vi "Un-Subscribe.vi"() -> ()   [LabVIEW 2013, in "FRCts20_SNS.lvlib"]
uses:
  FRCts20_SNS.lvlib
  Perforce/penguin_1666/mblack_PerforceWin/lvdotcom/source/aws-toolkit/r1/trunk/SNS/VI Source/AWS SNS Class/AWS_SNS.lvclass
  <vilib>/National Instruments/LabVIEW Interface for Amazon S3/Typedefs/AMZ_S3_AWS Credentials.ctl
  <vilib>/National Instruments/LabVIEW Interface for Amazon S3/LV Interface for Amazon S3.lvlib
  Perforce/penguin_1666/mblack_PerforceWin/lvdotcom/source/aws-toolkit/r1/trunk/SNS/VI Source/Public Typedefs/AWS_SNS Subcribe Parameters.ctl
  Perforce/penguin_1666/mblack_PerforceWin/lvdotcom/source/aws-toolkit/r1/trunk/SNS/VI Source/AWS_SNS.lvlib
  Perforce/penguin_1666/mblack_PerforceWin/lvdotcom/source/aws-toolkit/r1/trunk/SNS/VI Source/Public Typedefs/AWS_SNS Subscription.ctl
  Perforce/penguin_1666/mblack_PerforceWin/lvdotcom/source/aws-toolkit/r1/trunk/SNS/VI Source/Response Typedefs/ListSubscriptionsByTopicResult.ctl
panel:
  out "ListSubscriptions Result":T1
  in  "Event Name":string
  in  "Cell#":string
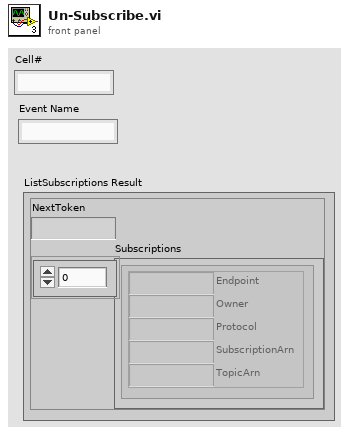
[diagram p1: front panel]
types:
  T1 = typedef "AWS_SNS.lvlib/ListSubscriptionsByTopicResult.ctl" = cluster{"NextToken":string, "Subscriptions":T2[]}
  T2 = typedef "AWS_SNS.lvlib/AWS_SNS Subscription.ctl" = cluster{"Endpoint":string, "Owner":string, "Protocol":string, "SubscriptionArn":string, "TopicArn":string}
  T3 = typedef "AWS_SNS.lvlib/AWS_SNS Subcribe Parameters.ctl" = cluster{"Endpoint":string, "Protocol":string, "TopicArn":string}
  T4 = typedef "LV Interface for Amazon S3.lvlib/AMZ_S3_AWS Credentials.ctl" = cluster{"Access Key":string, "Secret Key":string}
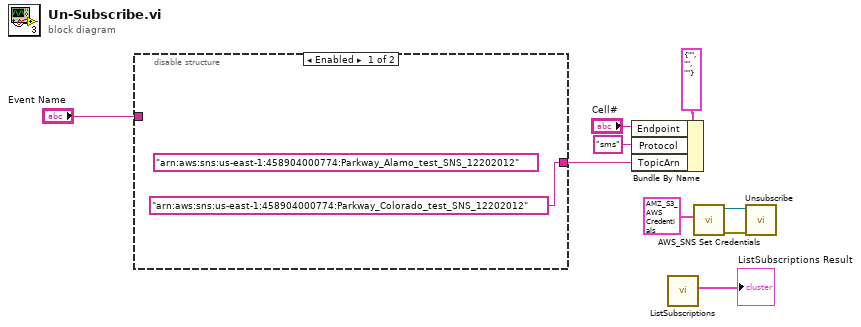
[diagram p0: block diagram]
diagram:
  n1 = disable-structure shown="Enabled" {
    disable-tunnel: ["arn:aws:sns:us-east-1:458904000774:Parkway_Colorado_test_SNS_12202012" ("TopicArn") _] -> w2
    disable-tunnel: "Event Name" -> [_ _]
    frame Enabled {
      (unwired) "arn:aws:sns:us-east-1:458904000774:Parkway_Alamo_test_SNS_12202012" ("TopicArn")
    }
    frame Disabled {
    }
  }
  n2 = Bundle By Name(cluster=T3 {"Endpoint"="", "Protocol"="", "TopicArn"=""} ("Subscribe Parameters"), "Endpoint"="Cell#", "Protocol"="sms", "TopicArn"=w2) -> ()  [unwired: 1 out]
  n3 = call-dynamic "ListSubscriptions.vi"() -> ("ListSubscriptions Result"=→"ListSubscriptions Result":T1)  [unwired: 9 in, 2 out]
  n4 = call "AWS_SNS Set Credentials.vi"("AWS Credentials"=T4 {"Access Key"="AKIAI4UOFGXQQ2XM3KTQ", "Secret Key"="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"} ("AWS Credentials in")) -> ("error out"=w3:errorcluster, "AWS_SNS.lvlib:AWS_SNS.lvclass"=w4:refnum<class "AWS_SNS.lvclass">)  [unwired: 9 in]
  n5 = call-dynamic "Unsubscribe.vi"("error in (no error)"=w3, "AWS_SNS.lvlib:AWS_SNS.lvclass"=w4) -> ()  [unwired: 8 in, 2 out]
